vi "prompt_and_enter_value2.vi"(10 "prompt_IN":string, 11 "Enter value":dbl) -> (3 "Numeric":dbl format="%.2f")   [LabVIEW 2016]
panel:
  out "prompt":string="HEIGHT FROM GROUND SURFACE TO SAMPLE BOX\n\nMeasure the vertical distance between the ground surface and the pressure transducer."
  in  "OK Button":bool
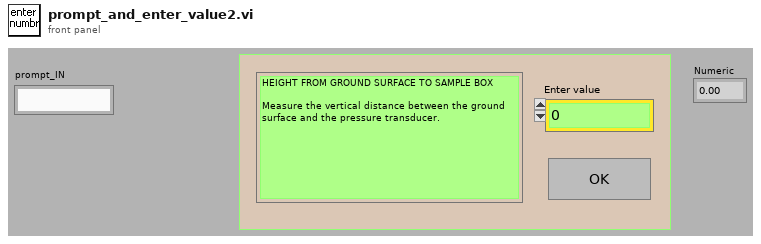
[diagram p1: front panel]
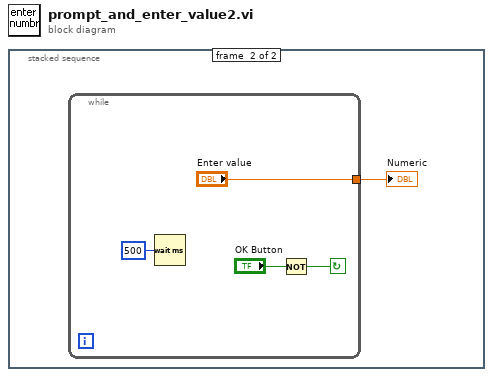
[diagram p0: block diagram]
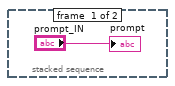
[diagram p2: hidden frame]
diagram:
  n1 = stacked-sequence {
    frame #0 {
      "prompt" <- "prompt_IN"
    }
    frame #1 {
      n2 = while {
        tunnel: ["Enter value"] -> w2
        stop <- w5 continue-if-true
        n3 = Wait (ms)(milliseconds to wait=u32 500) -> ()  [unwired: 1 out]
        n4 = Not(x="OK Button") -> (.not. x?=w5:bool)
      }
      "Numeric" <- w2
    }
  }
